vi "worker loop.vi"(8 "results reporter":refnum<class "results reporter.lvclass">, 9 "execution system":T1=enum."standard", 10 "thread pool":refnum<class "thread pool.lvclass">, 11 "communicator in":refnum<class "communicator.lvclass">) -> ()   [LabVIEW 2015, in "communicator.lvclass"]
uses:
  communicator.lvclass
  taskpool/dispatcher/thread pool.lvclass
  taskpool/dispatcher/execution system.ctl
  taskpool/results reporter/results reporter.lvclass
  message/communicator message.lvclass/communicator message.ctl
  communicator.lvclass/communicator.ctl
  communicator queue/identifying queue.lvclass/identifying queue.ctl
  message/create message.vi
  message/set sender.vi
  message/communicator message.lvclass
  communicator queue/identifying queue.lvclass
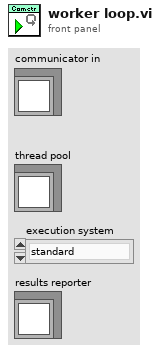
[diagram p1: front panel]
types:
  T1 = typedef "thread pool.lvclass/execution system.ctl" = enum32{"user interface", "standard", "instrument i/o", "data acquisition", "other 1", "other 2"}
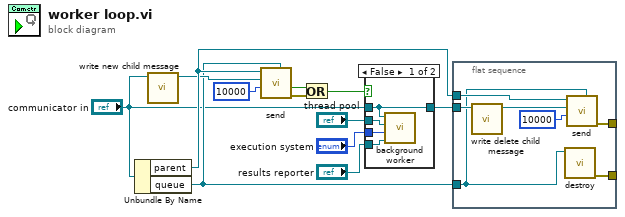
[diagram p0: block diagram]
diagram:
  n1 = Unbundle By Name("communicator in") -> ("parent"=w12:refnum<class "identifying queue.lvclass">, "queue"=w5:refnum<class "identifying queue.lvclass">)
  n2 = call "write new child message.vi"("child"="communicator in") -> ("message"=w10:refnum<class "communicator message.lvclass">)  [unwired: 10 in]
  n3 = call "send.vi"("sender"=w5, "timeout in ms (-1)"=10000, "message"=w10, "message connection in"=w12) -> ("error out"=w9:errorcluster, "timed out?"=w6:bool)  [unwired: 6 in]
  n4 = Or(x=w6, y=w9) -> (x .or. y?=w7:bool)
  n5 = case shown="False" w7 {
    tunnel: "communicator in" -> [w16 w17]
    tunnel: [w16 w17] -> w8
    tunnel: "thread pool" -> [w15 _]
    tunnel: "execution system" -> [w14 _]
    tunnel: "results reporter" -> [w13 _]
    frame False {
      n6 = call-dynamic "background worker.vi"("results reporter"=w13, "execution system"=w14, "thread pool"=w15, "communicator in"=w16) -> ()  [unwired: 8 in]
    }
    frame True {
    }
  }
  n7 = flat-sequence {
    tunnel: w12 -> [w24]
    tunnel: w8 -> [w21]
    tunnel: w5 -> [w18]
    tunnel: [w20] -> _
    tunnel: [w19] -> _
    frame #0 {
      n8 = call "write delete child message.vi"("child"=w21) -> ("message"=w23:refnum<class "communicator message.lvclass">)  [unwired: 10 in]
      n9 = call "destroy.vi"("message connection in"=w18) -> ("error out"=w19:errorcluster)  [unwired: 10 in]
      n10 = call "send.vi"("sender"=w18, "timeout in ms (-1)"=10000, "message"=w23, "message connection in"=w24) -> ("error out"=w20:errorcluster)  [unwired: 6 in, 1 out]
    }
  }
